vi "Teleop.vi"(10 "Match Info":T1={"Autonomous Elapsed Seconds"=0.0, "TeleOp Elapsed Seconds"=0.0, "Disabled Elapsed Seconds"=0.0, "Visited Autonomous"=FALSE, "Visited TeleOp"=FALSE, "Visited Disabled"=FALSE, "Autonomous Settings"={"Autonomous Style"=enum."Independent", "VI Refnum"=refnum}}, 11 "Call Context":T2) -> ()   [LabVIEW 2016]
doc: "This VI is called for each TeleOp packet received from the DS where the robot is not disabled. It is often used to read from the joysticks and update I/O or to update setpoints for timed control loops. It should complete and return within 20 milliseconds or it may miss DS packets."
uses:
  <vilib>/Rock Robotics/WPI/DriverStation/WPI_DriverStationDerivedRobotMode.ctl
  <vilib>/Rock Robotics/WPI/DriverStation/WPI_DriverStationMatch Info.ctl
  <vilib>/Rock Robotics/WPI/ThirdParty/Sensors/navX/_TypeDefs/FRIC_navX_DeviceNumbersTypeDef.ctl
  <vilib>/Rock Robotics/WPI/Solenoid/WPI_SolenoidValue.ctl
  <vilib>/Rock Robotics/Network Tables/NT Read Boolean.vi
  <vilib>/Rock Robotics/Network Tables/NT Read Number.vi
  <vilib>/Rock Robotics/WPI/Utilities/WPI_GetSetVariantRefNum.vi
  <vilib>/Rock Robotics/WPI/Solenoid/Deprecated/WPI_SolenoidSetBool.vi
  <vilib>/Rock Robotics/Network Tables/NT Write Number.vi
  <vilib>/Rock Robotics/WPI/Solenoid/WPI_SolenoidSetEnum.vi
panel:
  out "Distance 2":dbl
  out "Distance":dbl
  out "Sample Slider 0":dbl(slide) scale=0.0..5.0
  out "Sample Boolean 1":bool
  out "Sample Boolean 0":bool
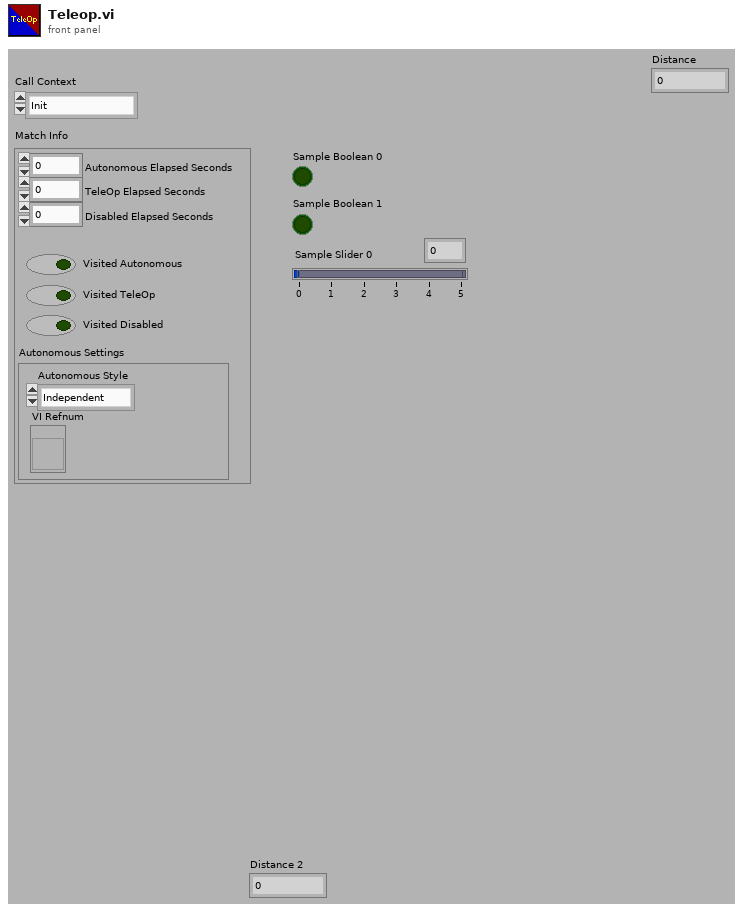
[diagram p1: front panel]
types:
  T1 = typedef "WPI_DriverStationMatch Info.ctl" = cluster{"Autonomous Elapsed Seconds":dbl, "TeleOp Elapsed Seconds":dbl, "Disabled Elapsed Seconds":dbl, "Visited Autonomous":bool, "Visited TeleOp":bool, "Visited Disabled":bool, "Autonomous Settings":cluster{"Autonomous Style":enum16{"Iterative", "Independent"}, "VI Refnum":refnum<vi>}}
  T2 = typedef "WPI_DriverStationDerivedRobotMode.ctl" = enum16{"Init", "Execute", "Stop"}
  T3 = typedef "FRIC_navX_DeviceNumbersTypeDef.ctl" = enum16{"Dev0", "Dev1", "Dev2", "Dev3"}
  T4 = typedef "WPI_EncoderDevRef.ctl" = cluster{"DevStatus":errorcluster, "EncoderIndex":T5, "CounterIndex":T6, "DistancePerCount":dbl, "Decoding Type":T7}
  T5 = typedef "FPGA_EncoderIdx.ctl" = enum8{"Enc 0", "Enc 1", "Enc 2", "Enc 3", "Enc 4", "Enc 5", "Enc 6", "Enc 7", "Invalid"}
  T6 = typedef "FPGA_CounterCtrSystemIndex.ctl" = enum8{"Ctr 0", "Ctr 1", "Ctr 2", "Ctr 3", "Ctr 4", "Ctr 5", "Ctr 6", "Ctr 7", "Invalid"}
  T7 = typedef "WPI_EncoderType.ctl" = enum16{"1x", "2x", "4x"}
  T8 = typedef "WPI_JoystickDevRef.ctl" = cluster{"Device":T9}
  T9 = typedef "WPI_JoystickDeviceEnum.ctl" = enum16{"USB 0", "USB 1", "USB 2", "USB 3", "USB 4", "USB 5"}
  T10 = typedef "WPI_MotorControlDeviceRef.ctl" = cluster{"DeviceStatus":errorcluster, "Type":T11, "PWM":cluster{"PWM Channel":T12, "DeadBand":T13}, "CAN":cluster{"Device Number":u8, "SetOutput VI Ref":variant, "GetOutput VI Ref":variant, "Enable VI Ref":variant, "Disable VI Ref":variant, "Data":variant}, "Invert":bool}
  T11 = typedef "WPI_MotorControlType.ctl" = enum16{"PWM", "CAN"}
  T12 = typedef "FPGA_DIOPWMChannel.ctl" = enum8{"PWM 0", "PWM 1", "PWM 2", "PWM 3", "PWM 4", "PWM 5", "PWM 6", "PWM 7", "PWM 8", "PWM 9", "PWM MXP 0", "PWM MXP 1", "PWM MXP 2", "PWM MXP 3", "PWM MXP 4", "PWM MXP 5", "PWM MXP 6", "PWM MXP 7", "PWM MXP 8", "PWM MXP 9", "Invalid"}
  T13 = typedef "WPI_PWMDeadband.ctl" = cluster{"Name":string, "maxPositivePwm":i32, "minPositivePwm":i32, "centerPwm":i32, "maxNegativePwm":i32, "minNegativePwm":i32, "angularRange":u16}
  T14 = typedef "WPI_RobotDriveDevRef.ctl" = cluster{"DevStatus":errorcluster, "Motors[]":T10[], "Square Inputs":bool, "Max Output":dbl}
  T15 = typedef "WPI_CompressorDevRef.ctl" = cluster{"DevStatus":errorcluster, "Pneumatics Control Module":u8}
  T16 = cluster{"Yaw":dbl, "Roll":dbl, "Pitch":dbl, "Heading":dbl, "Fused Heading":dbl}
  T17 = typedef "WPI_SolenoidDevRef.ctl" = cluster{"DevStatus":errorcluster, "Pneumatics Control Module":u8, "Forward Solenoid Channel":T18, "Reverse Solenoid Channel":T18}
  T18 = typedef "WPI_SolenoidChannel.ctl" = enum8{"Solenoid 0", "Solenoid 1", "Solenoid 2", "Solenoid 3", "Solenoid 4", "Solenoid 5", "Solenoid 6", "Solenoid 7", "Invalid"}
  T19 = typedef "WPI_SolenoidValue.ctl" = enum16{"Off", "On", "Forward", "Reverse"}
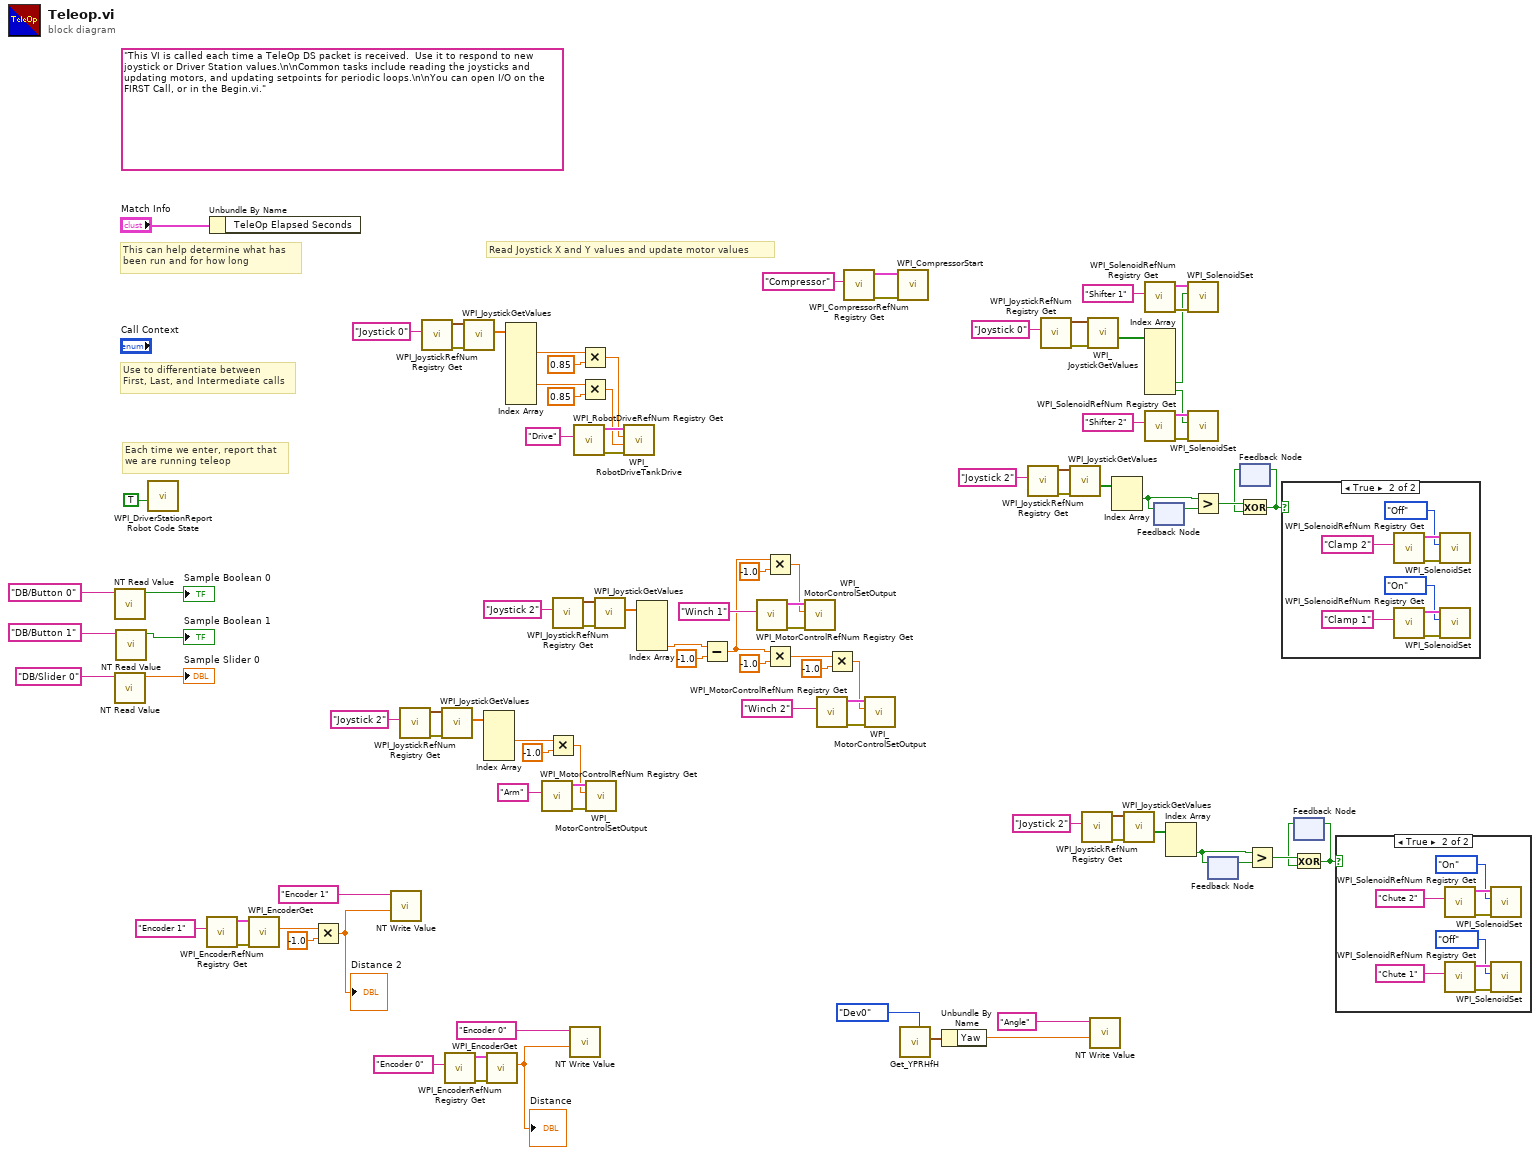
[diagram p0: block diagram]
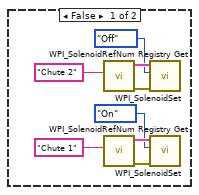
[diagram p2: hidden frame]
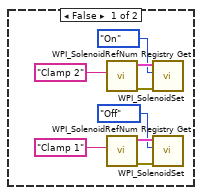
[diagram p3: hidden frame]
diagram:
  (unwired) "This VI is called each time a TeleOp DS packet is received.  Use it to respond to new joystick or Driver Station values.\n\nCommon tasks include reading the joysticks and updating motors, and updating setpoints for periodic loops.\n\nYou can open I/O on the FIRST Call, or in the Begin.vi."
  # "Each time we enter, report that\nwe are running teleop"
  # "Use to differentiate between\nFirst, Last, and Intermediate calls"
  # "This can help determine what has\nbeen run and for how long"
  # "Read Joystick X and Y values and update motor values"
  n1 = call-poly <vilib>:"NT Read Value.vi"("Name"="DB/Button 0" ("refnum name")) -> ("Boolean"=→"Sample Boolean 0":bool)  [unwired: 9 in, 1 out]
  n2 = call-poly <vilib>:"NT Read Value.vi"("Name"="DB/Slider 0" ("refnum name")) -> ("Numeric"=→"Sample Slider 0":dbl)  [unwired: 9 in, 1 out]
  n3 = call-poly <vilib>:"NT Read Value.vi"("Name"="DB/Button 1" ("refnum name")) -> ("Boolean"=→"Sample Boolean 1":bool)  [unwired: 9 in, 1 out]
  n4 = call <vilib>:"WPI_DriverStationReport Robot Code State.vi"("TeleOp"=TRUE ("Autonomous")) -> ()  [unwired: 10 in, 1 out]
  n5 = call <vilib>:"WPI_EncoderRefNum Registry Get.vi"("refnum name"="Encoder 1") -> ("error out"=w21:errorcluster, "EncoderDevRef"=w20:T4)  [unwired: 9 in]
  n6 = Unbundle By Name("Match Info") -> ()  [unwired: 1 out]
  n7 = call <vilib>:"WPI_EncoderGet.vi"("error in (no error)"=w21, "EncoderDevRef"=w20) -> ("Distance"=w14:dbl)  [unwired: 4 in, 5 out]
  n8 = Multiply(x=w14, y=-1.0) -> (x*y=w13:dbl)
  "Distance 2" <- w13
  n9 = call-poly <vilib>:"NT Write Value.vi"("Numeric"=w13, "Name"="Encoder 1") -> ()  [unwired: 9 in, 1 out]
  n10 = call <vilib>:"WPI_JoystickRefNum Registry Get.vi"("refnum name"="Joystick 2") -> ("error out"=w53:errorcluster, "JoystickDevRef"=w52:T8)  [unwired: 9 in]
  n11 = call <vilib>:"WPI_JoystickRefNum Registry Get.vi"("refnum name"="Joystick 0") -> ("error out"=w91:errorcluster, "JoystickDevRef"=w90:T8)  [unwired: 9 in]
  n12 = call <vilib>:"WPI_JoystickGetValues.vi"("error in (no error)"=w53, "JoystickDevRef"=w52) -> ("Axes"=w50:dbl[])  [unwired: 5 in, 4 out]
  n13 = call <vilib>:"WPI_EncoderRefNum Registry Get.vi"("refnum name"="Encoder 0") -> ("error out"=w24:errorcluster, "EncoderDevRef"=w23:T4)  [unwired: 9 in]
  n14 = call <vilib>:"WPI_JoystickGetValues.vi"("error in (no error)"=w91, "JoystickDevRef"=w90) -> ("Axes"=w88:dbl[])  [unwired: 5 in, 4 out]
  n15 = Index Array(array=w50) -> (element #2=w49:dbl)  [unwired: 4 in, 3 out]
  n16 = call <vilib>:"WPI_EncoderGet.vi"("error in (no error)"=w24, "EncoderDevRef"=w23) -> ("Distance"=w18:dbl)  [unwired: 4 in, 5 out]
  "Distance" <- w18
  n17 = Index Array(array=w88) -> (element #2=w2:dbl, element #6=w4:dbl)  [unwired: 8 in, 6 out]
  n18 = call <vilib>:"WPI_MotorControlRefNum Registry Get.vi"("refnum name"="Arm") -> ("error out"=w46:errorcluster, "MotorControlDevRef"=w47:T10)  [unwired: 9 in]
  n19 = Multiply(x=w49, y=-1.0) -> (x*y=w44:dbl)
  n20 = call <vilib>:"WPI_JoystickRefNum Registry Get.vi"("refnum name"="Joystick 2") -> ("error out"=w84:errorcluster, "JoystickDevRef"=w83:T8)  [unwired: 9 in]
  n21 = call-poly <vilib>:"NT Write Value.vi"("Numeric"=w18, "Name"="Encoder 0") -> ()  [unwired: 9 in, 1 out]
  n22 = call <vilib>:"WPI_RobotDriveRefNum Registry Get.vi"("refnum name"="Drive") -> ("error out"=w86:errorcluster, "RobotDriveDevRef"=w87:T14)  [unwired: 9 in]
  n23 = Multiply(x=w2, y=0.85) -> (x*y=w1:dbl)
  n24 = Multiply(x=w4, y=0.85) -> (x*y=w5:dbl)
  n25 = call <vilib>:"WPI_MotorControlSetOutput.vi"("error in (no error)"=w46, "Output"=w44, "MotorControlDevRef"=w47) -> ()  [unwired: 6 in, 3 out]
  n26 = call <vilib>:"WPI_JoystickGetValues.vi"("error in (no error)"=w84, "JoystickDevRef"=w83) -> ("Axes"=w81:dbl[])  [unwired: 5 in, 4 out]
  n27 = call <vilib>:"WPI_RobotDriveTankDrive.vi"("error in (no error)"=w86, "Right axis value"=w5, "Left axis value"=w1, "RobotDriveDevRef"=w87) -> ()  [unwired: 5 in, 3 out]
  n28 = Index Array(array=w81) -> (element #4=w73:dbl)  [unwired: 4 in, 3 out]
  n29 = Subtract(x=w73, y=-1.0) -> (x-y=w69:dbl)
  n30 = call <vilib>:"WPI_MotorControlRefNum Registry Get.vi"("refnum name"="Winch 1") -> ("error out"=w80:errorcluster, "MotorControlDevRef"=w79:T10)  [unwired: 9 in]
  n31 = Multiply(x=w69, y=-1.0) -> (x*y=w70:dbl)
  n32 = Multiply(x=w69, y=-1.0) -> (x*y=w54:dbl)
  n33 = call <vilib>:"WPI_MotorControlSetOutput.vi"("error in (no error)"=w80, "Output"=w70, "MotorControlDevRef"=w79) -> ()  [unwired: 6 in, 3 out]
  n34 = call <vilib>:"WPI_MotorControlRefNum Registry Get.vi"("refnum name"="Winch 2") -> ("error out"=w77:errorcluster, "MotorControlDevRef"=w76:T10)  [unwired: 9 in]
  n35 = Multiply(x=w54, y=-1.0) -> (x*y=w55:dbl)
  n36 = call <vilib>:"WPI_CompressorRefNum Registry Get.vi"("refnum name"="Compressor") -> ("error out"=w58:errorcluster, "CompressorDevRef"=w59:T15)  [unwired: 9 in]
  n37 = call <vilib>:"WPI_MotorControlSetOutput.vi"("error in (no error)"=w77, "Output"=w55, "MotorControlDevRef"=w76) -> ()  [unwired: 6 in, 3 out]
  n38 = call <vilib>:"WPI_CompressorStart.vi"("error in (no error)"=w58, "CompressorDevRef"=w59) -> ()  [unwired: 8 in, 2 out]
  n39 = call <vilib>:"Get_YPRHfH.vi"("Device Number"=FRIC_navX_DeviceNumbersTypeDef."Dev0") -> ("YRPHfH"=w11:T16)  [unwired: 10 in]
  n40 = Unbundle By Name(w11) -> ("Yaw"=w10:dbl)
  n41 = call <vilib>:"WPI_JoystickRefNum Registry Get.vi"("refnum name"="Joystick 2") -> ("error out"=w68:errorcluster, "JoystickDevRef"=w67:T8)  [unwired: 9 in]
  n42 = call <vilib>:"WPI_JoystickRefNum Registry Get.vi"("refnum name"="Joystick 0") -> ("error out"=w43:errorcluster, "JoystickDevRef"=w42:T8)  [unwired: 9 in]
  n43 = call <vilib>:"WPI_JoystickGetValues.vi"("error in (no error)"=w68, "JoystickDevRef"=w67) -> ("Buttons"=w65:bool[])  [unwired: 5 in, 4 out]
  n44 = call <vilib>:"WPI_JoystickRefNum Registry Get.vi"("refnum name"="Joystick 2") -> ("error out"=w33:errorcluster, "JoystickDevRef"=w32:T8)  [unwired: 9 in]
  n45 = call <vilib>:"WPI_JoystickGetValues.vi"("error in (no error)"=w43, "JoystickDevRef"=w42) -> ("Buttons"=w40:bool[])  [unwired: 5 in, 4 out]
  n46 = call-poly <vilib>:"NT Write Value.vi"("Numeric"=w10, "Name"="Angle") -> ()  [unwired: 9 in, 1 out]
  n47 = Index Array(array=w65) -> (element #1=w63:bool)  [unwired: 2 in, 1 out]
  n48 = call <vilib>:"WPI_JoystickGetValues.vi"("error in (no error)"=w33, "JoystickDevRef"=w32) -> ("Buttons"=w30:bool[])  [unwired: 5 in, 4 out]
  n49 = call <vilib>:"WPI_SolenoidRefNum Registry Get.vi"("refnum name"="Shifter 1") -> ("error out"=w39:errorcluster, "SolenoidDevRef"=w38:T17)  [unwired: 9 in]
  n50 = Index Array(array=w40) -> (element #5=w8:bool, element #6=w7:bool)  [unwired: 6 in, 4 out]
  n51 = call <vilib>:"WPI_SolenoidRefNum Registry Get.vi"("refnum name"="Shifter 2") -> ("error out"=w36:errorcluster, "SolenoidDevRef"=w35:T17)  [unwired: 9 in]
  n52 = feedback #1() -> (w64:bool)  [unwired: 1 in]
  n53 = feedback-in #1(w63) -> ()
  n54 = Index Array(array=w30) -> (element #2=w25:bool)  [unwired: 2 in, 1 out]
  n55 = call-poly <vilib>:"WPI_SolenoidSet.vi"("error in (no error)"=w39, "Value"=w8, "SolenoidDevRef"=w38) -> ()  [unwired: 7 in, 2 out]
  n56 = call-poly <vilib>:"WPI_SolenoidSet.vi"("error in (no error)"=w36, "Value"=w7, "SolenoidDevRef"=w35) -> ()  [unwired: 7 in, 2 out]
  n57 = Greater?(x=w63, y=w64) -> (0:w62:bool)
  n58 = feedback #2() -> (w29:bool)  [unwired: 1 in]
  n59 = feedback-in #2(w25) -> ()
  n60 = feedback #3() -> (w61:bool)  [unwired: 1 in]
  n61 = Exclusive Or(1:w61, 2:w62) -> (0:w60:bool)
  n62 = feedback-in #3(w60) -> ()
  n63 = Greater?(x=w25, y=w29) -> (0:w28:bool)
  n64 = case shown="True" w60 {
    frame False {
      n65 = call <vilib>:"WPI_SolenoidRefNum Registry Get.vi"("refnum name"="Clamp 2") -> ("error out"=w107:errorcluster, "SolenoidDevRef"=w106:T17)  [unwired: 9 in]
      n66 = call <vilib>:"WPI_SolenoidRefNum Registry Get.vi"("refnum name"="Clamp 1") -> ("error out"=w104:errorcluster, "SolenoidDevRef"=w103:T17)  [unwired: 9 in]
      n67 = call-poly <vilib>:"WPI_SolenoidSet.vi"("error in (no error)"=w107, "Value"=WPI_SolenoidValue."On", "SolenoidDevRef"=w106) -> ()  [unwired: 7 in, 2 out]
      n68 = call-poly <vilib>:"WPI_SolenoidSet.vi"("error in (no error)"=w104, "Value"=WPI_SolenoidValue."Off", "SolenoidDevRef"=w103) -> ()  [unwired: 7 in, 2 out]
    }
    frame True {
      n69 = call <vilib>:"WPI_SolenoidRefNum Registry Get.vi"("refnum name"="Clamp 2") -> ("error out"=w115:errorcluster, "SolenoidDevRef"=w114:T17)  [unwired: 9 in]
      n70 = call <vilib>:"WPI_SolenoidRefNum Registry Get.vi"("refnum name"="Clamp 1") -> ("error out"=w112:errorcluster, "SolenoidDevRef"=w111:T17)  [unwired: 9 in]
      n71 = call-poly <vilib>:"WPI_SolenoidSet.vi"("error in (no error)"=w115, "Value"=WPI_SolenoidValue."Off", "SolenoidDevRef"=w114) -> ()  [unwired: 7 in, 2 out]
      n72 = call-poly <vilib>:"WPI_SolenoidSet.vi"("error in (no error)"=w112, "Value"=WPI_SolenoidValue."On", "SolenoidDevRef"=w111) -> ()  [unwired: 7 in, 2 out]
    }
  }
  n73 = feedback #4() -> (w26:bool)  [unwired: 1 in]
  n74 = Exclusive Or(1:w26, 2:w28) -> (0:w27:bool)
  n75 = feedback-in #4(w27) -> ()
  n76 = case shown="True" w27 {
    frame False {
      n77 = call <vilib>:"WPI_SolenoidRefNum Registry Get.vi"("refnum name"="Chute 2") -> ("error out"=w123:errorcluster, "SolenoidDevRef"=w122:T17)  [unwired: 9 in]
      n78 = call <vilib>:"WPI_SolenoidRefNum Registry Get.vi"("refnum name"="Chute 1") -> ("error out"=w120:errorcluster, "SolenoidDevRef"=w119:T17)  [unwired: 9 in]
      n79 = call-poly <vilib>:"WPI_SolenoidSet.vi"("error in (no error)"=w123, "Value"=WPI_SolenoidValue."Off", "SolenoidDevRef"=w122) -> ()  [unwired: 7 in, 2 out]
      n80 = call-poly <vilib>:"WPI_SolenoidSet.vi"("error in (no error)"=w120, "Value"=WPI_SolenoidValue."On", "SolenoidDevRef"=w119) -> ()  [unwired: 7 in, 2 out]
    }
    frame True {
      n81 = call <vilib>:"WPI_SolenoidRefNum Registry Get.vi"("refnum name"="Chute 2") -> ("error out"=w131:errorcluster, "SolenoidDevRef"=w130:T17)  [unwired: 9 in]
      n82 = call <vilib>:"WPI_SolenoidRefNum Registry Get.vi"("refnum name"="Chute 1") -> ("error out"=w128:errorcluster, "SolenoidDevRef"=w127:T17)  [unwired: 9 in]
      n83 = call-poly <vilib>:"WPI_SolenoidSet.vi"("error in (no error)"=w131, "Value"=WPI_SolenoidValue."On", "SolenoidDevRef"=w130) -> ()  [unwired: 7 in, 2 out]
      n84 = call-poly <vilib>:"WPI_SolenoidSet.vi"("error in (no error)"=w128, "Value"=WPI_SolenoidValue."Off", "SolenoidDevRef"=w127) -> ()  [unwired: 7 in, 2 out]
    }
  }
